vi "Day 15-Astar.vi"(11 "Risk[n]":i32[][](array[numeric])) -> (1 "Goal":T1, 2 "cameFrom[n]":T1[][](array[typedef]), 3 "Minimum Risk Total":i32)   [LabVIEW 2021]
uses:
  <vilib>/Utility/miscctls.llb/LVMapReplaceAction.ctl
  Day 15-Position.ctl
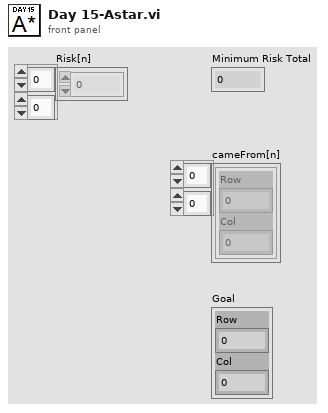
[diagram p1: front panel]
types:
  T1 = typedef "Day 15-Position.ctl" = cluster{"Row":i32, "Col":i32}
  T2 = typedef "LVMapReplaceAction.ctl" = enum32{"Modify Entry only if found", "Add or Modify Entry", "Delete Entry"}
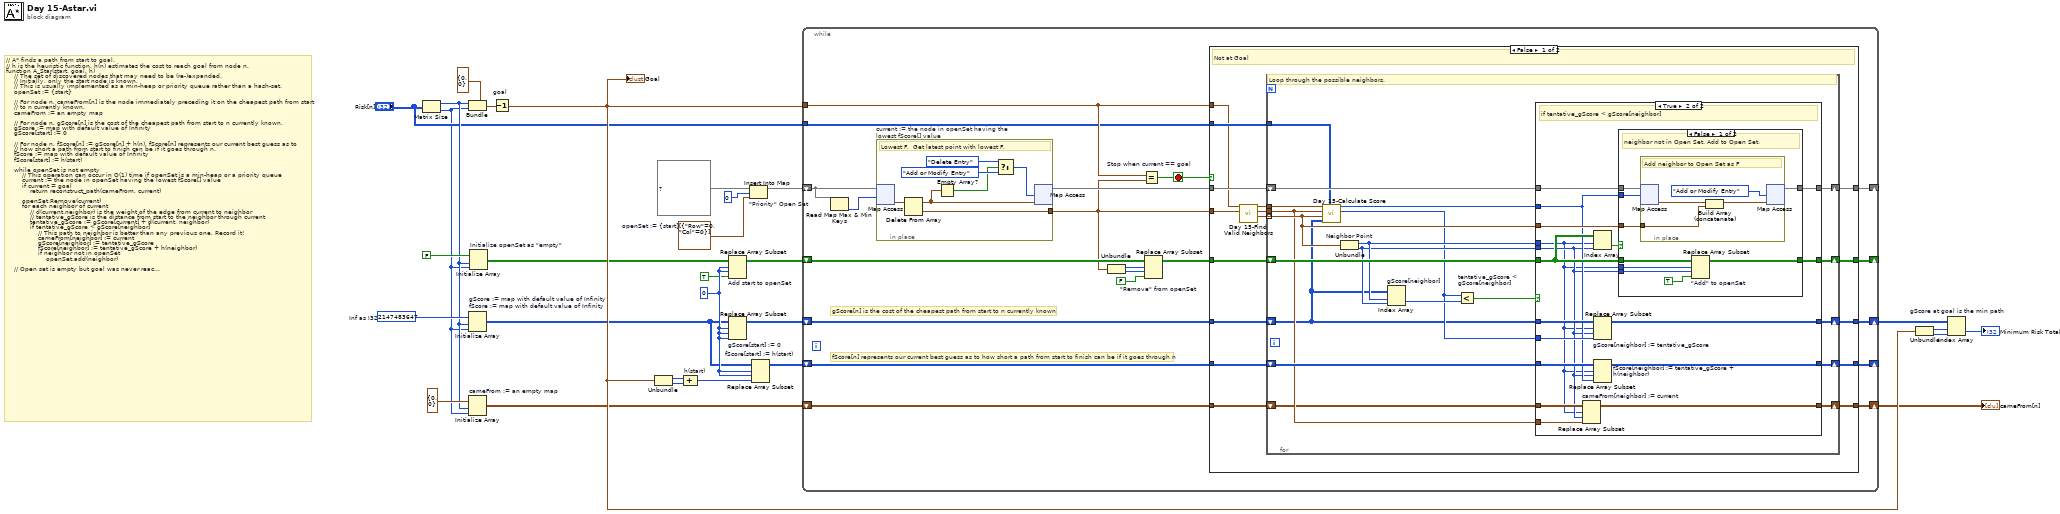
[diagram p0: block diagram]
diagram:
  w20 = 0 ("index (row)")
  w9 = 2147483647  # Inf as I32
  w8 = T1[] [{"Row"=0, "Col"=0}]  # openSet := {start}
  # "// A* finds a path from start to goal.\n// h is the heuristic function. h(n) estimates the cost to reach goal from node n.\nfunction A_Star(start, goal, h)\n    // The set of discovered nodes that may need to be (re-)expanded.\n    // Initially, only the start node is known.\n    // This is usually implemented as a min-heap or priority queue rather than a hash-set.\n    openSet := {start}\n\n    // For node n, cameFrom[n] is the node immediately preceding it on the cheapest path from start\n    // to n currently known.\n    cameFrom := an empty map\n\n    // For node n, gScore[n] is the cost of the cheapest path from start to n currently known.\n    gScore := map with default value of Infinity\n    gScore[start] := 0\n\n    // For node n, fScore[n] := gScore[n] + h(n). fScore[n] represents our current best guess as to\n    // how short a path from start to finish can be if it goes through n.\n    fScore := map with default value of Infinity\n    fScore[start] := h(start)\n\n    while openSet is not empty\n        // This operation can occur in O(1) time if openSet is a min-heap or a priority queue\n        current := the node in openSet having the lowest fScore[] value\n        if current = goal\n            return reconstruct_path(cameFrom, current)\n\n        openSet.Remove(current)\n        for each neighbor of current\n            // d(current,neighbor) is the weight of the edge from current to neighbor\n            // tentative_gScore is the distance from start to the neighbor through current\n            tentative_gScore := gScore[current] + d(current, neighbor)\n            if tentative_gScore < gScore[neighbor]\n                // This path to neighbor is better than any previous one. Record it!\n                cameFrom[neighbor] := current\n                gScore[neighbor] := tentative_gScore\n                fScore[neighbor] := tentative_gScore + h(neighbor)\n                if neighbor not in openSet\n                    openSet.add(neighbor)\n\n    // Open set is empty but goal was never reached\n    return failure"
  n1 = Matrix Size(0:"Risk[n]") -> (1:w3:i32, 2:w1:i32)
  n2 = Bundle(cluster=T1 {"Row"=0, "Col"=0} ("Position"), "Row"=w3, "Col"=w1) -> (w5:T1)
  n3 = Initialize Array "gScore := map with default value of Infinity\nfScore := map with default value of Infinity"(w9, w3, w1) -> (w19:i32[][])
  n4 = Initialize Array "cameFrom := an empty map"(T1 {"Row"=0, "Col"=0} ("Position"), w3, w1) -> (w27:T1[][])
  n5 = Initialize Array "Initialize openSet as \"empty\""(FALSE, w3, w1) -> (w13:bool[][])
  n6 = Decrement "goal"(x=w5) -> (x-1=w29:T1)
  "Goal" <- w29
  n7 = Unbundle(w29) -> ("Row"=w16:i32, "Col"=w17:i32)
  n8 = Compound Arithmetic op=ADD "h(start)"(w16, w17) -> (w21:i32)
  n9 = Replace Array Subset "Add start to openSet"(array=w13, new element=TRUE ("new element/subarray"), index (row)=w20, index (col)=w20) -> (w15:bool[][])
  n10 = Replace Array Subset "gScore[start] := 0"(array=w19, new element=w20, index (row)=w20, index (col)=w20) -> (w11:i32[][])
  n11 = Insert Into Map "\"Priority\" Open Set"(map in=map{i32, T1[]} {} ("Open Map"), key=0, value=w8) -> (map out=w10:map{i32, T1[]})  [unwired: 2 out]
  n12 = Replace Array Subset "fScore[start] := h(start)"(array=w19, new element=w21, index (row)=w20, index (col)=w20) -> (w18:i32[][])
  n13 = while {
    shift-right: [w45] -> _
    shift-left: w10 -> [w49]
    shift-right: [w43] -> w22
    shift-left: w11 -> [w44]
    tunnel: w29 -> [w42]
    shift-right: [w41] -> _
    shift-left: w15 -> [w40]
    shift-right: [w34] -> _
    shift-left: w18 -> [w33]
    tunnel: "Risk[n]" -> [w32]
    shift-right: [w30] -> w28
    shift-left: w27 -> [w31]
    stop <- w47 stop-if-true
    # "fScore[n] represents our current best guess as to how short a path from start to finish can be if it goes through n"
    # "gScore[n] is the cost of the cheapest path from start to n currently known"
    n14 = Read Map Max & Min Keys(11:w49) -> (1:w48:i32)  [unwired: 1 out]
    n15 = in-place "current := the node in openSet having the lowest fScore[] value" {
      in-place-border: [w55] -> w38
      # "Lowest F.  Get latest point with lowest F."
      n16 = in-place-map #1(w49, w48) -> (w56:T1[])  [unwired: 1 in, 1 out]
      n17 = Delete From Array(array=w56) -> (deleted portion=w55:T1, array with subset deleted=w54:T1[])  [unwired: 2 in]
      n18 = Empty Array?(array=w54) -> (empty?=w51:bool)
      n19 = Select(t=LVMapReplaceAction."Delete Entry" ("action"), s=w51, f=LVMapReplaceAction."Add or Modify Entry" ("action")) -> (s? t:f=w50:T2)
      n20 = in-place-map #1(w54, w50) -> (w46:map{i32, T1[]})  [unwired: 2 out]
    }
    n21 = Unbundle(w38) -> ("Row"=w37:i32, "Col"=w36:i32)
    n22 = Equal? "Stop when current == goal"(x=w42, y=w38) -> (x = y?=w47:bool)
    n23 = Replace Array Subset "\"Remove\" from openSet"(array=w40, new element=FALSE ("new element/subarray"), index (row)=w37, index (col)=w36) -> (w39:bool[][])
    n24 = case shown="False" w47 {
      tunnel: w46 -> [w71 w134]
      tunnel: [w69 w134] -> w45
      tunnel: w44 -> [w72 w133]
      tunnel: [w70 w133] -> w43
      tunnel: w38 -> [w60 _]
      tunnel: w42 -> [w62 _]
      tunnel: w39 -> [w68 w132]
      tunnel: [w67 w132] -> w41
      tunnel: [w66 w131] -> w34
      tunnel: w33 -> [w65 w131]
      tunnel: w32 -> [w64 _]
      tunnel: w31 -> [w58 w130]
      tunnel: [w57 w130] -> w30
      frame False {
        # "Not at Goal"
        n25 = call "Day 15-Find Valid Neighbors.vi"("Current in"=w60, "Goal in"=w62) -> ("All Neighbors"=w63:T1[], "Current out"=w59:T1, "Goal out"=w61:T1)  [unwired: 7 in]
        n26 = for {
          shift-right: [w84] -> w70
          shift-left: w72 -> [w74]
          shift-right: [w82] -> w69
          shift-left: w71 -> [w89]
          tunnel: w63 -> [w92] mode=indexing
          shift-right: [w83] -> w67
          shift-left: w68 -> [w88]
          shift-right: [w80] -> w66
          shift-left: w65 -> [w81]
          tunnel: w64 -> [w79]
          tunnel: w61 -> [w78]
          tunnel: w59 -> [w77]
          shift-right: [w75] -> w57
          shift-left: w58 -> [w76]
          # "Loop through the possible neighbors."
          n27 = call "Day 15-Calculate Score.vi"("Risk"=w79, "G"=w74, "Neighbor"=w92, "Current"=w77, "Goal"=w78) -> ("gScore(neighbor)"=w85:i32, "fScore(neighbor)"=w73:i32)  [unwired: 5 in]
          n28 = Unbundle "Neighbor Point"(w92) -> ("Row"=w87:i32, "Col"=w86:i32)
          n29 = Index Array "gScore[neighbor]"(array=w74, index (row)=w87, index (col)=w86) -> (element=w91:i32)
          n30 = Less? "tentative_gScore < \ngScore[neighbor]"(x=w85, y=w91) -> (x < y?=w90:bool)
          n31 = case shown="True" w90 {
            tunnel: w74 -> [w97 w109]
            tunnel: w89 -> [w95 w111]
            tunnel: w88 -> [w96 w113]
            tunnel: [w97 w107] -> w84
            tunnel: [w96 w112] -> w83
            tunnel: [w95 w110] -> w82
            tunnel: w87 -> [_ w98]
            tunnel: w86 -> [_ w99]
            tunnel: w85 -> [_ w108]
            tunnel: w73 -> [_ w103]
            tunnel: w92 -> [_ w106]
            tunnel: [w94 w105] -> w80
            tunnel: w81 -> [w94 w104]
            tunnel: w77 -> [_ w100]
            tunnel: w76 -> [w93 w101]
            tunnel: [w93 w102] -> w75
            frame False {
            }
            frame True {
              # "if tentative_gScore < gScore[neighbor]"
              n32 = Replace Array Subset "cameFrom[neighbor] := current"(array=w101, new element=w100, index (row)=w98, index (col)=w99) -> (w102:T1[][])
              n33 = Index Array(array=w113, index (row)=w98, index (col)=w99) -> (element=w114:bool)
              n34 = Replace Array Subset "gScore[neighbor] := tentative_gScore"(array=w109, new element=w108, index (row)=w98, index (col)=w99) -> (w107:i32[][])
              n35 = Replace Array Subset "fScore[neighbor] := tentative_gScore + h(neighbor)"(array=w104, new element=w103, index (row)=w98, index (col)=w99) -> (w105:i32[][])
              n36 = case shown="False" w114 {
                tunnel: w113 -> [w120 w129]
                tunnel: [w119 w129] -> w112
                tunnel: w111 -> [w123 w128]
                tunnel: [w121 w128] -> w110
                tunnel: w106 -> [w122 _]
                tunnel: w98 -> [w118 _]
                tunnel: w99 -> [w117 _]
                tunnel: w103 -> [w115 _]
                frame False {
                  # "neighbor not in Open Set. Add to Open Set."
                  n37 = in-place {
                    in-place-border: w122 -> [w126]
                    # "Add neighbor to Open Set as F"
                    n38 = in-place-map #2(w123, w115) -> (w125:T1[])  [unwired: 1 in, 1 out]
                    n39 = Build Array (concatenate)(w125, w126) -> (w124:T1[])
                    n40 = in-place-map #2(w124, LVMapReplaceAction."Add or Modify Entry" ("action")) -> (w121:map{i32, T1[]})  [unwired: 2 out]
                  }
                  n41 = Replace Array Subset "\"Add\" to openSet"(array=w120, new element=TRUE ("new element/subarray"), index (row)=w118, index (col)=w117) -> (w119:bool[][])
                }
                frame True {
                  # "neighbor is in Open Set"
                }
              }
            }
          }
        }
      }
      frame True {
        # "Reached Goal"
      }
    }
  }
  "cameFrom[n]" <- w28
  n42 = Unbundle(w29) -> ("Row"=w23:i32, "Col"=w24:i32)
  n43 = Index Array "gScore at goal is the min path"(array=w22, index (row)=w23, index (col)=w24) -> (element=→"Minimum Risk Total":i32)
